vi "GetControlSize.vi"(9 "Control in":refnum<class "Control.lvclass">) -> (3 "Control out":refnum<class "Control.lvclass">, 4 "size":cluster{"x":i16, "y":i16})   [LabVIEW 2014, in "Raspberry Pi Compatible Compiler for LabVIEW.lvlib" / "Control.lvclass"]
uses:
  Control.lvclass
  GObject/GObject.lvclass/GObject.ctl
  GObject/GObject.lvclass
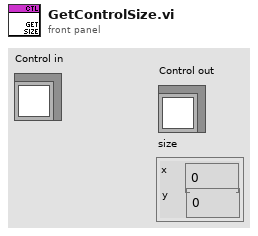
[diagram p1: front panel]
types:
  T1 = typedef "LVRectTypeDef.ctl" = cluster{"Left":i16, "Top":i16, "Right":i16, "Bottom":i16}
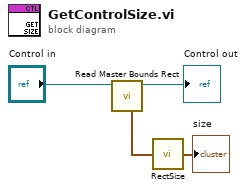
[diagram p0: block diagram]
diagram:
  n1 = call "Read Master Bounds Rect.vi"("GObject in"="Control in") -> ("GObject out"=→"Control out":refnum<class "Control.lvclass">, "Master Bounds Rect"=w3:T1)  [unwired: 7 in]
  n2 = call <vilib>:"RectSize.vi"("rect"=w3) -> ("point"=→"size":cluster{"x":i16, "y":i16})
